vi "PH_PPPA_PowerUnit.Event Calls for Reset.vi"(0 "i ref in":refnum<vi>, 3 "PU":T1, 5 "error in (no error)":errorcluster) -> (14 "i ref out":refnum<vi>, 19 "error out":errorcluster)   [LabVIEW 2014, in "PH_PPPA_PowerUnit.lvlib"]
doc: "This VI is necessary to reset a DEL PSU (or others?) after a sum fault occured."
uses:
  PH_PPPA_PowerUnit.lvlib
  PH_Basics/PH_PP_Common/PH_PP_Common.PUs.ctl
  PH_Devices/PH_Beckhoff_PP_PU/PH_Beckhoff_PP_PU.lvlib
  PH_Basics/PH_PP_Common/PH_PP_Common.lvlib
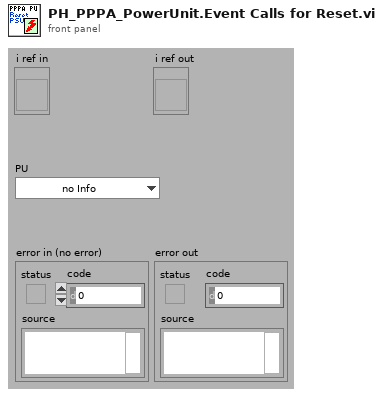
[diagram p1: front panel]
types:
  T1 = typedef "PH_PP_Common.lvlib/PH_PP_Common.PUs.ctl" = enum16{"no Info", "PA-19mm-1", "PA-19mm-2", "PA-45mm-PILC", "PA-45mm-MAIN", "MA-PU-1", "MA-PU-2", "MA-PU-3", "MA-PU-4", "MA-PU-5", "MA-PU-6", "MA-FR", "MA-PILC", "PA-45mm-DP"}
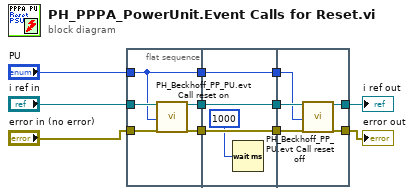
[diagram p0: block diagram]
diagram:
  n1 = flat-sequence {
    tunnel: "error in (no error)" -> [w16]
    tunnel: "i ref in" -> [w14]
    tunnel: "PU" -> [w12]
    tunnel: [w15] -> w11
    tunnel: [w13] -> w10
    tunnel: [w12] -> w9
    tunnel: w11 -> [w20]
    tunnel: w10 -> [w19]
    tunnel: [w20] -> w8
    tunnel: [w19] -> w7
    tunnel: [w17] -> w6
    tunnel: w9 -> [w17]
    tunnel: [w22] -> w3
    tunnel: [w24] -> w4
    tunnel: w8 -> [w25]
    tunnel: w7 -> [w23]
    tunnel: w6 -> [w21]
    frame #0 {
      n2 = call "PH_Beckhoff_PP_PU.evt Call reset on.vi"("i ref in"=w14, "PU"=w12, "error in"=w16) -> ("i ref out"=w13:refnum<vi>, "error out"=w15:errorcluster)  [unwired: 15 in]
    }
    frame #1 {
      n3 = Wait (ms)(milliseconds to wait=u32 1000) -> ()  [unwired: 1 out]
    }
    frame #2 {
      n4 = call "PH_Beckhoff_PP_PU.evt Call reset off.vi"("i ref in"=w23, "PU"=w21, "error in"=w25) -> ("i ref out"=w22:refnum<vi>, "error out"=w24:errorcluster)  [unwired: 15 in]
    }
  }
  "error out" <- w4
  "i ref out" <- w3
